vi "VoltageCfg.vi"(8 "error in (no error)":errorcluster, 10 "Vertical Settings":T1={"ChannelSelection"=enum."chn A", "Coupling"=0, "Offset[V]"=0.0, "V/div"=4.0} {"V/div" scale=0.0..6.0; "Coupling" items=["AC", "DC"]}, 11 "reference in":refnum<k24>) -> (0 "error out":errorcluster, 1 "Setup Info Vertical":T5, 3 "reference out":refnum<k24>)   [LabVIEW 2019, in "LabNation Scope Driver.lvlib"]
doc: "Sets up the Gain, Coupling and Offset of the Smart Scope."
uses:
  LabNation Scope Driver.lvlib
  C:/Program Files (x86)/LabNation/SmartScope/DeviceInterface.dll
  Program Files (x86)/LabNation/SmartScope/DeviceInterface.dll
  Typedef/Metadata/[Meta]SetupInfoV.ctl
  Typedef/Channel Selection.ctl
  Typedef/Vertical Settings.ctl
  Typedef/Coupling.ctl
  Typedef/RangeSetting.ctl
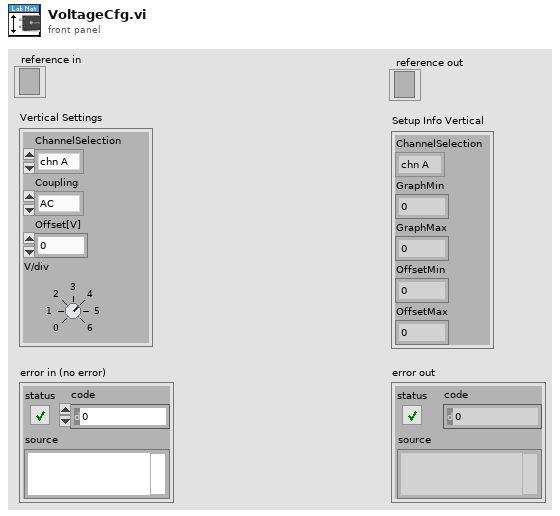
[diagram p1: front panel]
types:
  T1 = typedef "LabNation Scope Driver.lvlib/Vertical Settings.ctl" = cluster{"ChannelSelection":T2, "Coupling":T3, "Offset[V]":dbl, "V/div":T4}
  T2 = typedef "LabNation Scope Driver.lvlib/Channel Selection.ctl" = enum16{"chn A", "chn B"}
  T3 = typedef "LabNation Scope Driver.lvlib/Coupling.ctl" = i32
  T4 = typedef "LabNation Scope Driver.lvlib/RangeSetting.ctl" = dbl
  T5 = typedef "LabNation Scope Driver.lvlib/[Meta]SetupInfoV.ctl" = cluster{"ChannelSelection":T2, "GraphMin":dbl, "GraphMax":dbl, "OffsetMin":dbl, "OffsetMax":dbl}
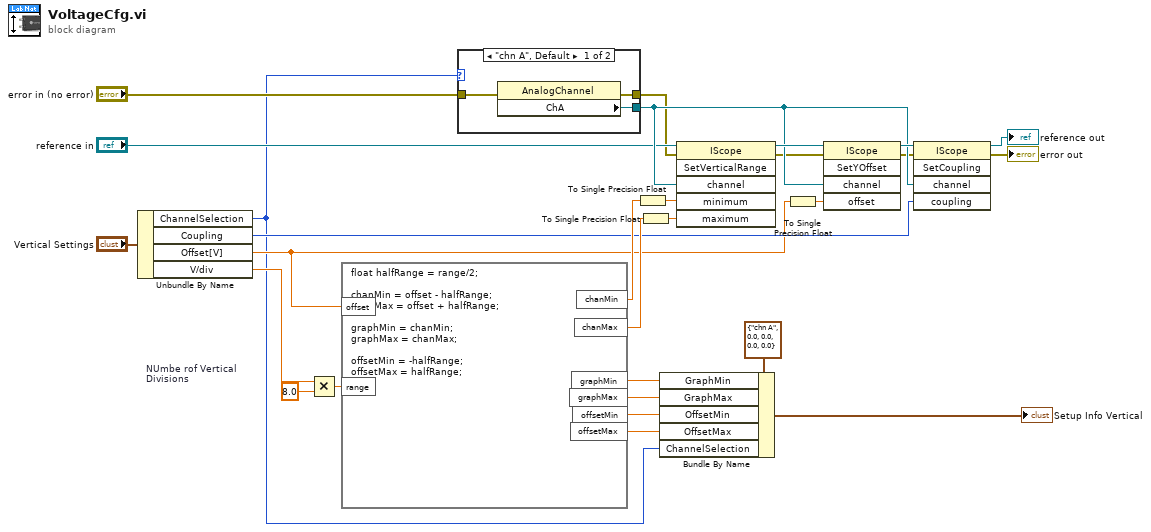
[diagram p0: block diagram]
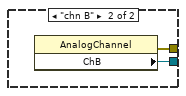
[diagram p2: hidden frame]
diagram:
  w4 = 8.0  # NUmbe rof Vertical Divisions
  n1 = Unbundle By Name("Vertical Settings") -> ("ChannelSelection"=w1:T2, "Coupling"=w11:T3, "Offset[V]"=w10:dbl, "V/div"=w2:T4)
  n2 = Multiply(x=w2, y=w4) -> (x*y=w3:T4)
  n3 = formula code="float halfRange = range/2;\n\nchanMin = offset - halfRange;\nchanMax = offset + halfRange;\n\ngraphMin = chanMin;\ngraphMax = chanMax;\n\noffsetMin = -halfRange;\noffsetMax = halfRange;"("range"=w3, "offset"=w10) -> ("chanMin"=w25:dbl, "chanMax"=w23:dbl, "offsetMin"=w14:dbl, "offsetMax"=w13:dbl, "graphMin"=w16:dbl, "graphMax"=w15:dbl)
  n4 = case shown="\"chn A\", Default" w1 {
    tunnel: [w31 w33] -> w21
    tunnel: [w30 w32] -> w7
    tunnel: "error in (no error)" -> [w29 _]
    frame "chn A", Default {
      n5 = property class="AnalogChannel"(error in=w29) -> (error out=w30:errorcluster, "ChA"=w31:refnum<k24>)  [unwired: 1 in, 1 out]
    }
    frame "chn B" {
      n6 = property class="AnalogChannel"() -> (error out=w32:errorcluster, "ChB"=w33:refnum<k24>)  [unwired: 2 in, 1 out]
    }
  }
  n7 = To Single Precision Float(number=w25) -> (single precision float=w26:sgl)
  n8 = To Single Precision Float(number=w23) -> (single precision float=w24:sgl)
  n9 = Bundle By Name(cluster=T5 {"ChannelSelection"=enum."chn A", "GraphMin"=0.0, "GraphMax"=0.0, "OffsetMin"=0.0, "OffsetMax"=0.0} ("Setup Info Vertical"), "GraphMin"=w16, "GraphMax"=w15, "OffsetMin"=w14, "OffsetMax"=w13, "ChannelSelection"=w1) -> (→"Setup Info Vertical":T5)
  n10 = invoke class="IScope" method="SetVerticalRange"(reference="reference in", error in=w7, "channel"=w21, "minimum"=w26, "maximum"=w24) -> (reference out=w27:refnum<k24>, error out=w6:errorcluster)  [unwired: 1 in, 4 out]
  n11 = To Single Precision Float(number=w10) -> (single precision float=w22:sgl)
  n12 = invoke class="IScope" method="SetYOffset"(reference=w27, error in=w6, "channel"=w21, "offset"=w22) -> (reference out=w28:refnum<k24>, error out=w5:errorcluster)  [unwired: 1 in, 3 out]
  n13 = invoke class="IScope" method="SetCoupling"(reference=w28, error in=w5, "channel"=w21, "coupling"=w11) -> (reference out=→"reference out":refnum<k24>, error out=→"error out":errorcluster)  [unwired: 1 in, 3 out]
